vi "Init - Add APU.vi"(8 "error in (no error)":errorcluster, 10 "APU Component":T2, 11 "Device ref in":T1 format="%.0x") -> (0 "error out":errorcluster, 3 "Device Ref out":T1 format="%.0x")   [LabVIEW 2011, in "Engine Sim System Explorer.lvlib"]
uses:
  Engine Sim System Explorer.lvlib
  <vilib>/NI Veristand/Custom Device API/Custom Device Item Ref.ctl
  TypeDefs/APUComp.ctl
  <vilib>/NI Veristand/Custom Device API/Custom Device Channel.ctl
  <vilib>/NI Veristand/Custom Device API/Custom Device Channel Type.ctl
  Shared/Engine Simulation Global.vi
  <vilib>/NI Veristand/Custom Device API/Set Item Property (Variant).vi
  <vilib>/NI Veristand/Custom Device API/Custom Device API.lvlib
  Engine Simulation Shared.lvlib
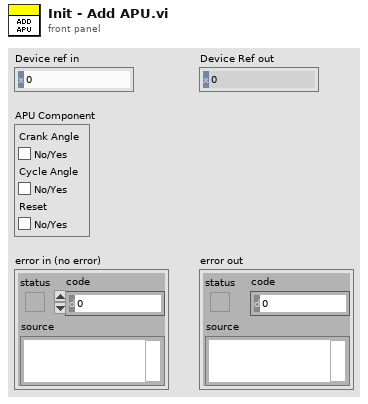
[diagram p1: front panel]
types:
  T1 = typedef "Custom Device API.lvlib/Custom Device Item Ref.ctl" = u64
  T2 = typedef "Engine Sim System Explorer.lvlib/APUComp.ctl" = cluster{"Crank Angle":bool, "Cycle Angle":bool, "Reset":bool}
  T3 = typedef "Custom Device API.lvlib/Custom Device Channel.ctl" = cluster{"Type":T4, "Units":string, "Default Value":dbl, "Faultable":bool, "Scalable":bool}
  T4 = typedef "Custom Device API.lvlib/Custom Device Channel Type.ctl" = enum16{"Input", "Output"}
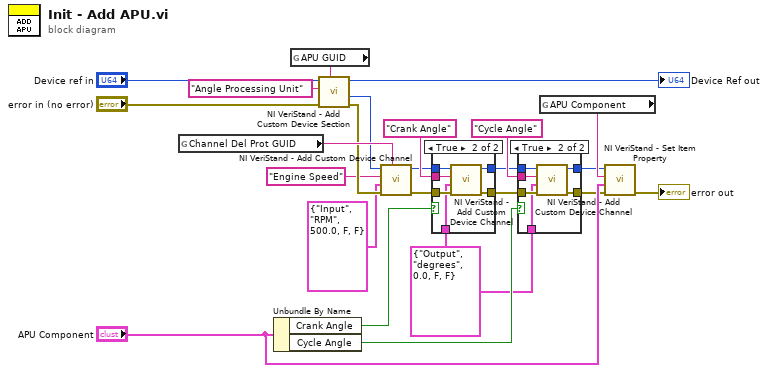
[diagram p0: block diagram]
diagram:
  w7 = T3 {"Type"=enum."Output", "Units"="degrees", "Default Value"=0.0, "Faultable"=FALSE, "Scalable"=FALSE} ("Channel")
  n1 = global read "Engine Simulation Global.vi" "Channel Del Prot GUID"() -> (w22:string)
  n2 = Unbundle By Name("APU Component") -> ("Crank Angle"=w12:bool, "Cycle Angle"=w13:bool)
  n3 = global read "Engine Simulation Global.vi" "APU GUID"() -> (w19:string)
  n4 = call <vilib>:"NI VeriStand - Add Custom Device Section.vi"("GUID (Default Section)"=w19, "error in (no error)"="error in (no error)", "Section Name"="Angle Processing Unit", "Parent Ref in"="Device ref in") -> ("error out"=w18:errorcluster, "Section Ptr"=w20:T1, "Parent Ref out"=→"Device Ref out":T1)  [unwired: 4 in, 1 out]
  n5 = call <vilib>:"NI VeriStand - Add Custom Device Channel.vi"("GUID (Default Channel)"=w22, "error in (no error)"=w18, "Channel"=T3 {"Type"=enum."Input", "Units"="RPM", "Default Value"=500.0, "Faultable"=FALSE, "Scalable"=FALSE}, "Channel Name"="Engine Speed", "Parent Ref in"=w20) -> ("error out"=w5:errorcluster, "Parent Ref out"=w6:T1)  [unwired: 3 in, 2 out]
  n6 = case shown="True" w12 {
    tunnel: w5 -> [w25 w32]
    tunnel: w6 -> [w26 w31]
    tunnel: [w25 w30] -> w9
    tunnel: [w26 w29] -> w8
    tunnel: w7 -> [_ w28]
    tunnel: "Crank Angle" ("Channel Name") -> [_ w27]
    frame False {
    }
    frame True {
      n7 = call <vilib>:"NI VeriStand - Add Custom Device Channel.vi"("error in (no error)"=w32, "Channel"=w28, "Channel Name"=w27, "Parent Ref in"=w31) -> ("error out"=w30:errorcluster, "Parent Ref out"=w29:T1)  [unwired: 4 in, 2 out]
    }
  }
  n8 = case shown="True" w13 {
    tunnel: w9 -> [w33 w40]
    tunnel: w8 -> [w34 w39]
    tunnel: [w33 w38] -> w14
    tunnel: [w34 w37] -> w15
    tunnel: w7 -> [_ w36]
    tunnel: "Cycle Angle" ("Channel Name") -> [_ w35]
    frame False {
    }
    frame True {
      n9 = call <vilib>:"NI VeriStand - Add Custom Device Channel.vi"("error in (no error)"=w40, "Channel"=w36, "Channel Name"=w35, "Parent Ref in"=w39) -> ("error out"=w38:errorcluster, "Parent Ref out"=w37:T1)  [unwired: 4 in, 2 out]
    }
  }
  n10 = global read "Engine Simulation Global.vi" "APU Component"() -> (w16:string)
  n11 = call-poly <vilib>:"NI VeriStand - Set Item Property.vi"("error in (no error)"=w14, "Value"="APU Component", "Property Name"=w16, "Item Ref in"=w15) -> ("error out"=→"error out":errorcluster)  [unwired: 5 in, 2 out]
